vi "4461 Export Triggers.vi"(8 "error in (no error)":errorcluster, 10 "master task in":refnum<k21>, 11 "task in":refnum<k21>) -> (0 "error out":errorcluster, 3 "task out":refnum<k21>)   [LabVIEW 2016, in "Lockin.DAQ.lvclass"]
uses:
  Lockin.DAQ.lvclass
  <vilib>/DAQmx/configure/trigger.llb/DAQmx Start Trigger (Digital Edge).vi
  <resource>/objmgr/daqmx.rc
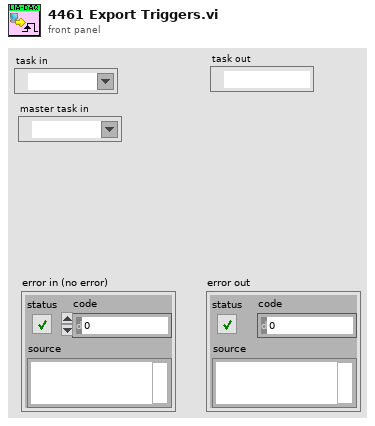
[diagram p1: front panel]
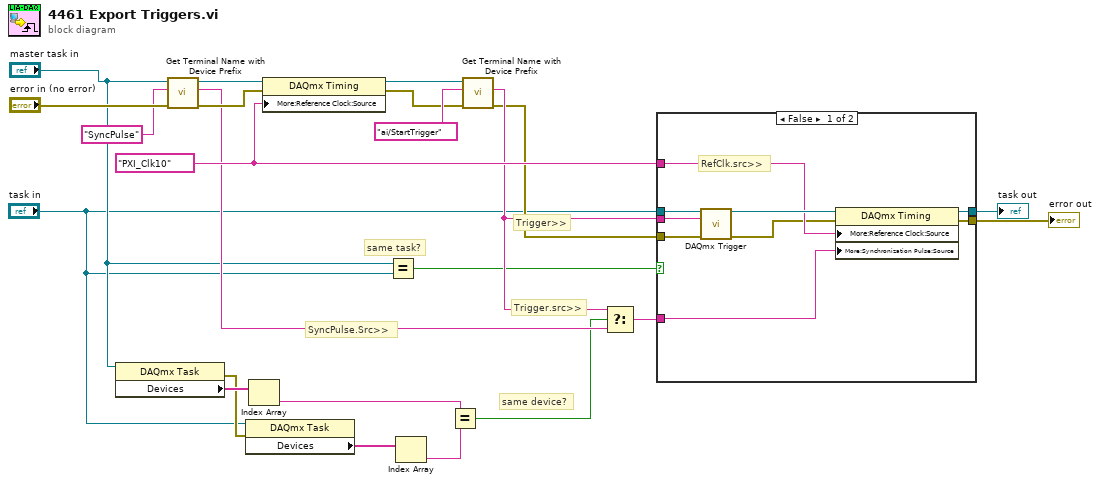
[diagram p0: block diagram]
diagram:
  w13 = tag "PXI_Clk10" ("RefClk.Src")
  # "same task?"
  # "SyncPulse.Src>>"
  # "same device?"
  # "Trigger>>"
  # "Trigger.src>>"
  n1 = property class="DAQmx Task"(reference="master task in") -> (error out=w6:errorcluster, "Devices"=w15:tag[])  [unwired: 1 in, 1 out]
  n2 = call "Get Terminal Name with Device Prefix.vi"("error in (no error)"="error in (no error)", "Local Terminal Name"="SyncPulse", "task/channels in"="master task in") -> ("error out"=w18:errorcluster, "Terminal Name with Device Prefix"=w11:tag, "task out"=w22:refnum<k21>)  [unwired: 6 in]
  n3 = property class="DAQmx Task"(reference="task in", error in=w6) -> ("Devices"=w14:tag[])  [unwired: 2 out]
  n4 = Index Array(array=w15) -> (element=w10:tag)  [unwired: 1 in]
  n5 = property class="DAQmx Timing"(reference=w22, error in=w18, "More:Reference Clock:Source"=w13) -> (reference out=w21:refnum<k21>, error out=w19:errorcluster)
  n6 = Equal?(x="master task in", y="task in") -> (x = y?=w1:bool)
  n7 = Index Array(array=w14) -> (element=w9:tag)  [unwired: 1 in]
  n8 = Equal?(x=w10, y=w9) -> (x = y?=w8:bool)
  n9 = call "Get Terminal Name with Device Prefix.vi"("error in (no error)"=w19, "Local Terminal Name"="ai/StartTrigger", "task/channels in"=w21) -> ("error out"=w7:errorcluster, "Terminal Name with Device Prefix"=w12:tag)  [unwired: 6 in, 1 out]
  n10 = Select(t=w12, s=w8, f=w11) -> (s? t:f=w16:tag)
  n11 = case shown="False" w1 {
    tunnel: w16 -> [w31 _]
    tunnel: w13 -> [w30 _]
    tunnel: w12 -> [w29 _]
    tunnel: w7 -> [w28 w33]
    tunnel: [w27 w34] -> w5
    tunnel: [w25 w33] -> w4
    tunnel: "task in" -> [w24 w34]
    frame False {
      # "RefClk.src>>"
      n12 = call-poly <vilib>:"DAQmx Trigger.vi"("task/channels in"=w24, "source"=w29, "error in"=w28) -> ("task out"=w32:refnum<k21>, "error out"=w26:errorcluster)  [unwired: 11 in]
      n13 = property class="DAQmx Timing"(reference=w32, error in=w26, "More:Reference Clock:Source"=w30, "More:Synchronization Pulse:Source"=w31) -> (reference out=w27:refnum<k21>, error out=w25:errorcluster)
    }
    frame True {
    }
  }
  "error out" <- w4
  "task out" <- w5
